vi "ImageButtonFacade.vi"(0 "Data In":T4, 2 "Display State In":T2 {"image" items=["Left", "LeftBig", "LeftSmall", "Right", "RightBig", "RightSmall", "Up", "UpBig", "UpSmall", "Down", "DownBig", "DownSmall", "Zero", "Play", "Pause", "Load", "Lower", "Raise", "Home", "Home2"]}, 3 "Container State":T3) -> (6 "Data Out":T4, 7 "Display State Out":T2 {"image" items=["Left", "LeftBig", "LeftSmall", "Right", "RightBig", "RightSmall", "Up", "UpBig", "UpSmall", "Down", "DownBig", "DownSmall", "Zero", "Play", "Pause", "Load", "Lower", "Raise", "Home", "Home2"]}, 8 "Action":T1)   [LabVIEW 2020, in "ImageButton2.xctl"]
uses:
  ImageButton2.xctl
  ImageButtonData.ctl
  <vilib>/_xctls/Container State.ctl
  ImageButtonState.ctl
  <vilib>/_xctls/Action.ctl
  C:/Projects/RaxTagServer/LabviewDXFViewer/LabviewDXFViewer/bin/Release/LabviewDXFViewer.exe
  LabviewDXFViewer/bin/Release/LabviewDXFViewer.exe
  <vilib>/_xctls/XControlSupport.lvlib
panel:
  in  "ImageButton":refnum<k24>(container)
types:
  T1 = typedef "XControlSupport.lvlib/Action.ctl" = cluster{"Data Changed?":bool, "State Changed?":bool, "Action Name":string}
  T2 = typedef "ImageButton2.xctl/ImageButtonState.ctl" = cluster{"image":i32}
  T3 = typedef "XControlSupport.lvlib/Container State.ctl" = cluster{"Indicator?":bool, "Run Mode?":bool, " Refnum":refnum<vi>}
  T4 = typedef "ImageButton2.xctl/ImageButtonData.ctl" = bool
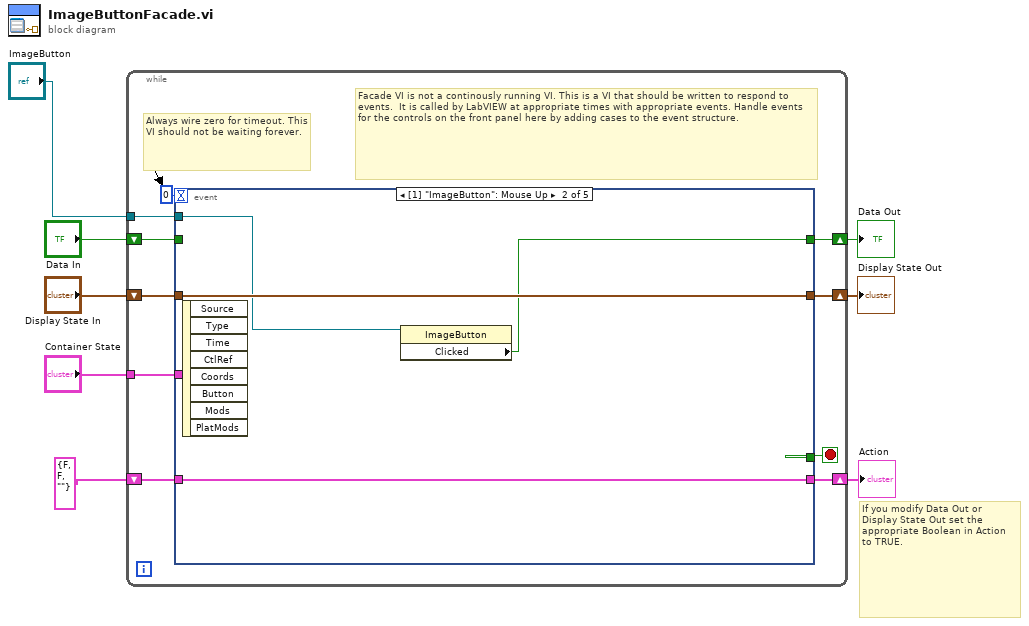
[diagram p0: block diagram]
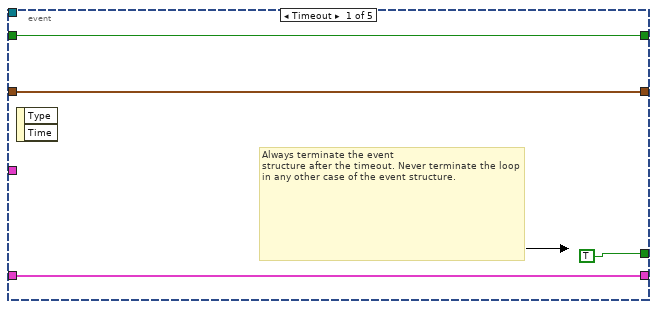
[diagram p2: hidden frame]
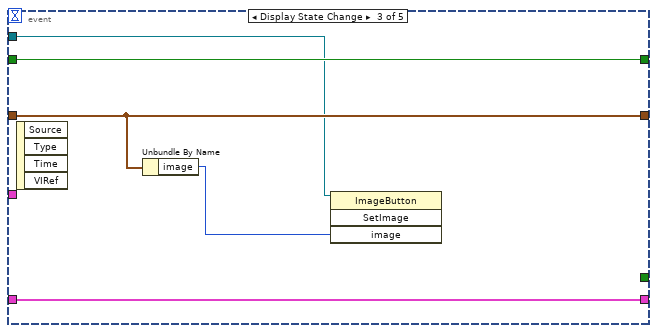
[diagram p3: hidden frame]
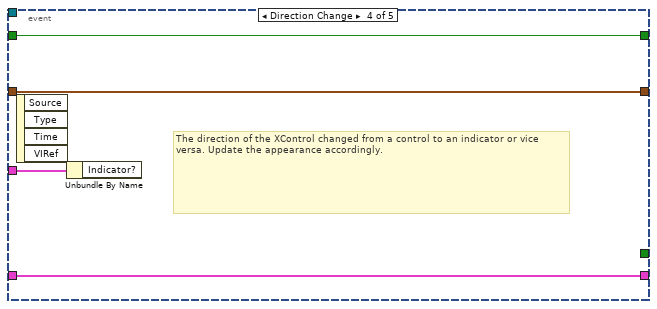
[diagram p4: hidden frame]
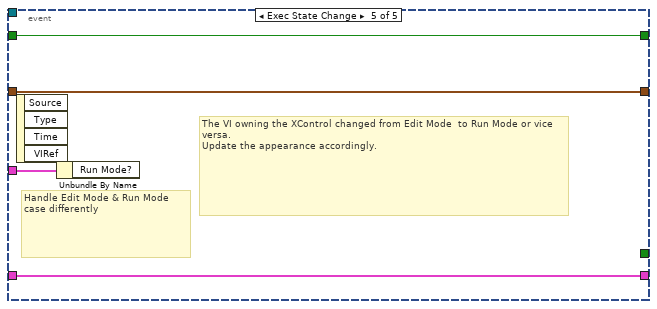
[diagram p5: hidden frame]
diagram:
  # "If you modify Data Out or\nDisplay State Out set the\nappropriate Boolean in Action\nto TRUE."
  n1 = while {
    shift-right: [w17] -> w5
    shift-left: "Display State In" -> [w18]
    tunnel: "Container State" -> [w14]
    shift-right: [w12] -> w8
    shift-left: "Data In" -> [w13]
    shift-right: [w10] -> w3
    shift-left: T1 {"Data Changed?"=FALSE, "State Changed?"=FALSE, "Action Name"=""} ("Action") -> [w11]
    tunnel: "ImageButton" -> [w9]
    stop <- w16 stop-if-true
    # "Facade VI is not a continously running VI. This is a VI that should be written to respond to events.  It is called by LabVIEW at appropriate times with appropriate events. Handle events for the controls on the front panel here by adding cases to the event structure."
    # "Always wire zero for timeout. This\nVI should not be waiting forever."
    n2 = event shown="[1] \"ImageButton\": Mouse Up" {
      selector: _ -> [_ _ _ _ _]
      dyn-events: _ -> [_ _ _ _ _]
      timeout: 0 -> [_ _ _ _ _]
      tunnel: w18 -> [w20 w26 w29 w34 w38]
      tunnel: [w20 w26 w29 w34 w38] -> w17
      tunnel: [TRUE _ _ _ _] -> w16
      tunnel: w14 -> [_ _ _ w35 w39]
      tunnel: w13 -> [w19 _ w31 w33 w37]
      tunnel: [w19 w23 w31 w33 w37] -> w12
      tunnel: [w21 w25 w30 w32 w36] -> w10
      tunnel: w11 -> [w21 w25 w30 w32 w36]
      tunnel: w9 -> [_ w24 w28 _ _]
      event Timeout {
        # "Always terminate the event\nstructure after the timeout. Never terminate the loop in any other case of the event structure."
        n3 = event-data() -> ()  [unwired: 1 in, 2 out]
      }
      event "ImageButton": Mouse Up {
        n4 = event-data() -> ()  [unwired: 1 in, 8 out]
        n5 = property class="ImageButton"(reference=w24) -> ("Clicked"=w23:bool)  [unwired: 1 in, 2 out]
      }
      event Display State Change {
        n6 = event-data() -> ()  [unwired: 1 in, 4 out]
        n7 = Unbundle By Name(w29) -> ("image"=w27:i32)
        n8 = invoke class="ImageButton" method="SetImage"(reference=w28, "image"=w27) -> ()  [unwired: 2 in, 4 out]
      }
      event Direction Change {
        # "The direction of the XControl changed from a control to an indicator or vice versa. Update the appearance accordingly."
        n9 = event-data() -> ()  [unwired: 1 in, 4 out]
        n10 = Unbundle By Name(w35) -> ()  [unwired: 1 out]
      }
      event Exec State Change {
        # "The VI owning the XControl changed from Edit Mode  to Run Mode or vice versa.\nUpdate the appearance accordingly."
        # "Handle Edit Mode & Run Mode\ncase differently"
        n11 = event-data() -> ()  [unwired: 1 in, 4 out]
        n12 = Unbundle By Name(w39) -> ()  [unwired: 1 out]
      }
    }
  }
  "Display State Out" <- w5
  "Data Out" <- w8
  "Action" <- w3
